vi "Read Response Content.vi"(8 "error in (no error)":errorcluster, 11 "HttpResponseMessage in":refnum<class "HttpResponseMessage.lvclass">) -> (0 "error out":errorcluster, 2 "HttpContent out":refnum<class "HttpContent.lvclass">, 3 "HttpResponseMessage out":refnum<class "HttpResponseMessage.lvclass">)   [LabVIEW 2018, in "HttpClient_NET.lvlib" / "HttpResponseMessage.lvclass"]
doc: "<b> </b> <b> </b>\nHttpClient_NET\nJustin Young - Viviota\nCopyright (c) 2021\nLicense: BSD"
uses:
  HttpResponseMessage.lvclass
  HttpContent/HttpContent.lvclass
  HttpResponseMessage.lvclass/HttpResponseMessage.ctl
  System.Net.Http
  Accessors/Write HttpContent.vi
  Accessors/Read NET_HttpReponseMessage.vi
  Accessors/Read HttpContent.vi
  Accessors/Read Timeout_ms.vi
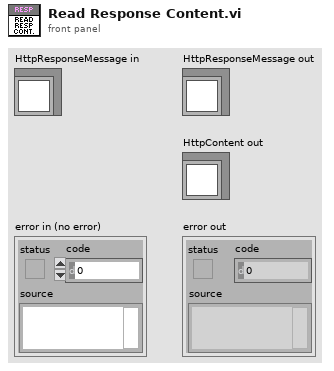
[diagram p1: front panel]
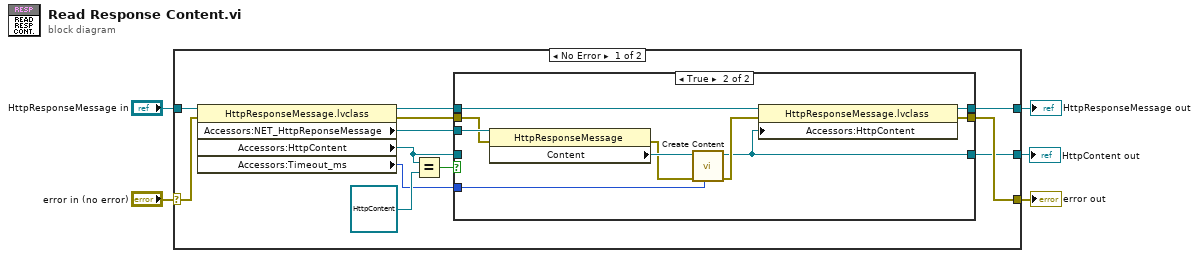
[diagram p0: block diagram]
diagram:
  n1 = case shown="No Error" "error in (no error)" {
    selector: "error in (no error)" -> [w17 w32]
    tunnel: [w13 w32] -> w4
    tunnel: [w11 w31] -> w2
    tunnel: "HttpResponseMessage in" -> [w16 w31]
    tunnel: [w10 _] -> w1
    frame No Error {
      n2 = property class="HttpResponseMessage.lvclass"(reference=w16, error in=w17) -> (reference out=w12:refnum<class "HttpResponseMessage.lvclass">, error out=w14:errorcluster, "Accessors:NET_HttpReponseMessage"=w15:refnum<k24>, "Accessors:HttpContent"=w7:refnum<class "HttpContent.lvclass">, "Accessors:Timeout_ms"=w6:i32)
      n3 = Equal?(x=w7, y=refnum<class "HttpContent.lvclass"> refnum) -> (x = y?=w8:bool)
      n4 = case shown="True" w8 {
        tunnel: w15 -> [_ w30]
        tunnel: w14 -> [w18 w28]
        tunnel: [w18 w25] -> w13
        tunnel: w12 -> [w19 w24]
        tunnel: [w19 w23] -> w11
        tunnel: [w20 w22] -> w10
        tunnel: w7 -> [w20 _]
        tunnel: w6 -> [_ w21]
        frame False {
        }
        frame True {
          n5 = property class="HttpResponseMessage"(reference=w30, error in=w28) -> (error out=w27:errorcluster, "Content"=w29:refnum<k24>)  [unwired: 1 out]
          n6 = call "Create Content.vi"("timeout_ms"=w21, "error in (no error)"=w27, "NET_HttpContent"=w29) -> ("error out"=w26:errorcluster, "HttpContent out"=w22:refnum<class "HttpContent.lvclass">)  [unwired: 7 in]
          n7 = property class="HttpResponseMessage.lvclass"(reference=w24, error in=w26, "Accessors:HttpContent"=w22) -> (reference out=w23:refnum<class "HttpResponseMessage.lvclass">, error out=w25:errorcluster)
        }
      }
    }
    frame Error {
    }
  }
  "error out" <- w4
  "HttpResponseMessage out" <- w2
  "HttpContent out" <- w1
